vi "Daemon_JETAbout Launcher.vi"(8 "error in":errorcluster, 9 "Dialog Text":string, 10 "Dialog Name":string, 11 "jModule":refnum<class "jModule.lvclass">) -> (0 "error out":errorcluster, 2 "VI Refnum":refnum<vi>, 3 "jModule":refnum<class "jModule.lvclass">)   [LabVIEW 2019]
doc: "This VI is used to launch the Daemon.\n\nIt also adds the Daemon to the jModule so that the jModule can manage shutting the deamon down in the event of a software shutdown.\nJSMA Module Template - Top Level UI 0.2.0.4\nRob Humfeld - Jet Engineering\nCopyright (c) 2019, Jet Engineering"
uses:
  <userlib>/Jet Engineering/JSMA/Libraries/jModule Class/jModule.lvclass
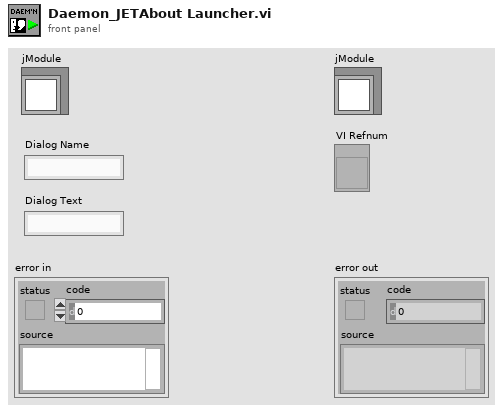
[diagram p1: front panel]
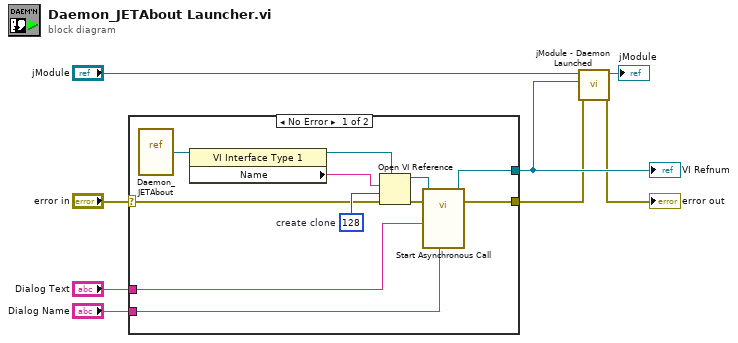
[diagram p0: block diagram]
diagram:
  n1 = case shown="No Error" "error in" {
    selector: "error in" -> [w11 w20]
    tunnel: [w18 w20] -> w1
    tunnel: [w12 _] -> w3
    tunnel: "Dialog Name" -> [w9 _]
    tunnel: "Dialog Text" -> [w10 _]
    frame No Error {
      w13 = 128  # create clone
      n2 = vi-ref "Daemon_JETAbout.vi"() -> (w17:refnum<vi>)
      n3 = property class="VI Interface Type 1"(reference=w17) -> (reference out=w16:refnum<vi>, "Name"=w14:string)  [unwired: 1 in, 1 out]
      n4 = Open VI Reference(type specifier VI Refnum (for type only)=w16, vi path=w14, options=w13, error in (no error)=w11) -> (vi reference=w15:refnum<vi>, error out=w19:errorcluster)  [unwired: 2 in]
      n5 = call-by-ref "Start Asynchronous Call"(reference=w15, error in=w19, "Dialog Name"=w9, "Dialog Parameters"=w10) -> (reference out=w12:refnum<vi>, error out=w18:errorcluster)  [unwired: 10 in]
    }
    frame Error {
    }
  }
  "VI Refnum" <- w3
  n6 = call <userlib>:"jModule - Daemon Launched.vi"("error in (no error)"=w1, "vi reference"=w3, "jModule"="jModule") -> ("error out"=→"error out":errorcluster, "jModule"=→"jModule":refnum<class "jModule.lvclass">)  [unwired: 6 in, 1 out]
